vi "Get Config.vi"(6 "?":T1=enum."path", 8 "error in (no error)":errorcluster, 9 "section":string, 10 "key":string, 11 "FileConfig in":refnum<class "FileConfig.lvclass">) -> (0 "error out":errorcluster, 1 "found?":bool, 2 "Data":variant, 3 "FileConfig out":refnum<class "FileConfig.lvclass">)   [LabVIEW 2019, in "Config.lvlib" / "FileConfig.lvclass"]
uses:
  FileConfig.lvclass
  Config/Controls/KeyType.ctl
  FileConfig.lvclass/FileConfig.ctl
  <vilib>/Utility/config.llb/Read Key (Boolean).vi
  <vilib>/Utility/config.llb/Read Key (I32).vi
  <vilib>/Utility/config.llb/Read Key (U32).vi
  <vilib>/Utility/config.llb/Read Key (String).vi
  <vilib>/Utility/config.llb/Read Key (Path).vi
  <vilib>/Utility/config.llb/Read Key (Double).vi
  Config.lvclass
  <vilib>/Utility/config.llb/NI_LVConfig.lvlib
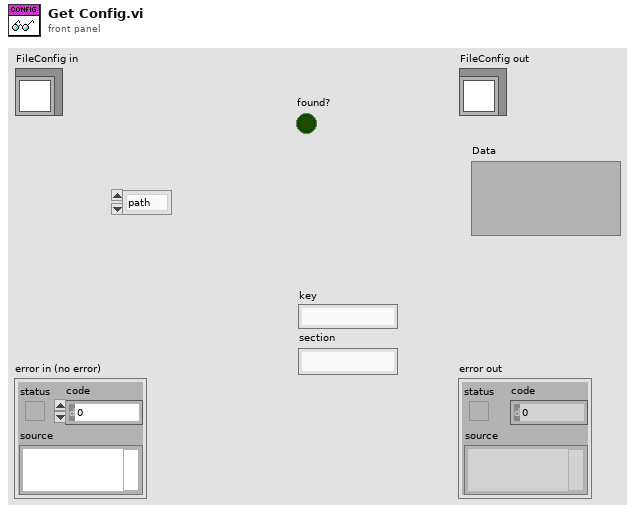
[diagram p1: front panel]
types:
  T1 = typedef "Config.lvlib/Config.lvclass/KeyType.ctl" = enum16{"dbl", "path", "string ", "u32", "i32", "boolean"}
  T2 = typedef "NI_LVConfig.lvlib/Config Data RefNum.ctl" = refnum<k1>
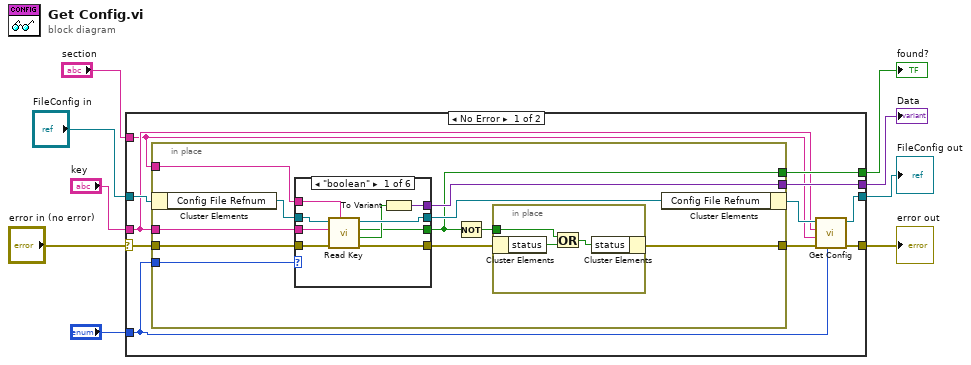
[diagram p0: block diagram]
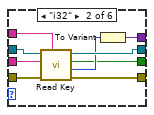
[diagram p2: hidden frame]
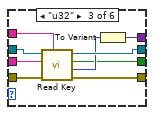
[diagram p3: hidden frame]
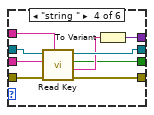
[diagram p4: hidden frame]
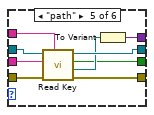
[diagram p5: hidden frame]
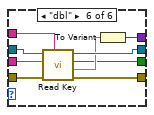
[diagram p6: hidden frame]
diagram:
  n1 = case shown="No Error" "error in (no error)" {
    selector: "error in (no error)" -> [w16 w90]
    tunnel: [w19 w90] -> w8
    tunnel: "FileConfig in" -> [w18 w89]
    tunnel: [w20 w89] -> w6
    tunnel: "?" -> [w12 _]
    tunnel: "key" -> [w11 _]
    tunnel: "section" -> [w10 _]
    tunnel: [w14 _] -> w2
    tunnel: [w13 _] -> w1
    frame No Error {
      n2 = in-place {
        in-place-border: w11 -> [w31]
        in-place-border: w10 -> [w30]
        in-place-border: w16 -> [w27]
        in-place-border: [w22] -> w15
        in-place-border: [w24] -> w14
        in-place-border: [w26] -> w13
        in-place-border: w12 -> [w25]
        n3 = in-place-cluster #1(w18) -> ("Config File Refnum"=w28:T2)
        n4 = case shown="\"boolean\"" w25 {
          tunnel: [w43 w51 w60 w70 w79 w87] -> w23
          tunnel: [w42 w52 w61 w69 w78 w88] -> w29
          tunnel: [w40 w49 w58 w67 w76 w86] -> w26
          tunnel: [w39 w48 w57 w66 w75 w84] -> w24
          tunnel: w31 -> [w37 w46 w55 w64 w74 w83]
          tunnel: w30 -> [w38 w47 w56 w65 w73 w82]
          tunnel: w28 -> [w36 w45 w54 w63 w72 w81]
          tunnel: w27 -> [w35 w44 w53 w62 w71 w80]
          frame "boolean" {
            n5 = call-poly <vilib>:"Read Key.vi"("section"=w38, "error in (no error)"=w35, "key"=w37, "refnum"=w36) -> ("error out"=w43:errorcluster, "value"=w41:bool, "found?"=w39:bool, "refnum out"=w42:T2)  [unwired: 4 in]
            n6 = To Variant(anything=w41) -> (Variant=w40:variant)
          }
          frame "i32" {
            n7 = call-poly <vilib>:"Read Key.vi"("section"=w47, "error in (no error)"=w44, "key"=w46, "refnum"=w45) -> ("error out"=w51:errorcluster, "value"=w50:i32, "found?"=w48:bool, "refnum out"=w52:T2)  [unwired: 4 in]
            n8 = To Variant(anything=w50) -> (Variant=w49:variant)
          }
          frame "u32" {
            n9 = call-poly <vilib>:"Read Key.vi"("section"=w56, "error in (no error)"=w53, "key"=w55, "refnum"=w54) -> ("error out"=w60:errorcluster, "value"=w59:u32, "found?"=w57:bool, "refnum out"=w61:T2)  [unwired: 4 in]
            n10 = To Variant(anything=w59) -> (Variant=w58:variant)
          }
          frame "string " {
            n11 = call-poly <vilib>:"Read Key.vi"("section"=w65, "error in (no error)"=w62, "key"=w64, "refnum"=w63) -> ("error out"=w70:errorcluster, "value"=w68:string, "found?"=w66:bool, "refnum out"=w69:T2)  [unwired: 4 in]
            n12 = To Variant(anything=w68) -> (Variant=w67:variant)
          }
          frame "path" {
            n13 = call-poly <vilib>:"Read Key.vi"("section"=w73, "error in (no error)"=w71, "key"=w74, "refnum"=w72) -> ("error out"=w79:errorcluster, "value"=w77:path, "found?"=w75:bool, "refnum out"=w78:T2)  [unwired: 4 in]
            n14 = To Variant(anything=w77) -> (Variant=w76:variant)
          }
          frame "dbl" {
            n15 = call-poly <vilib>:"Read Key.vi"("section"=w82, "error in (no error)"=w80, "key"=w83, "refnum"=w81) -> ("error out"=w87:errorcluster, "value"=w85:dbl, "found?"=w84:bool, "refnum out"=w88:T2)  [unwired: 4 in]
            n16 = To Variant(anything=w85) -> (Variant=w86:variant)
          }
        }
        n17 = Not(x=w24) -> (.not. x?=w21:bool)
        n18 = in-place {
          in-place-border: w21 -> [w34]
          n19 = in-place-cluster #2(w23) -> ("status"=w32:bool)
          n20 = Or(x=w34, y=w32) -> (x .or. y?=w33:bool)
          n21 = in-place-cluster #2("status"=w33) -> (w22:errorcluster)
        }
        n22 = in-place-cluster #1("Config File Refnum"=w29) -> (w17:refnum<class "FileConfig.lvclass">)
      }
      n23 = call-parent "Get Config.vi"(6:w12, "error in (no error)"=w15, "section"=w10, "key"=w11, "Config in"=w17) -> ("error out"=w19:errorcluster, "Config out"=w20:refnum<class "FileConfig.lvclass">)  [unwired: 3 in, 2 out]
    }
    frame Error {
    }
  }
  "error out" <- w8
  "FileConfig out" <- w6
  "Data" <- w1
  "found?" <- w2
